vi "Exit Processing.vi"(8 "error in (no error)":errorcluster, 11 "InteractionProcessor in":refnum<class "InteractionProcessor.lvclass">) -> (0 "error out":errorcluster)   [LabVIEW 2023, in "HAF.lvlib" / "InteractionProcessor.lvclass"]
doc: "Processing will exit. Ensure a clean shutdown. All Commands are asked to cleanup which performs a controlled shutdown of Drivers."
uses:
  InteractionProcessor.lvclass
  CommandDirector/CommandDirector.lvclass
  WriteCommand/WriteCommand.lvclass
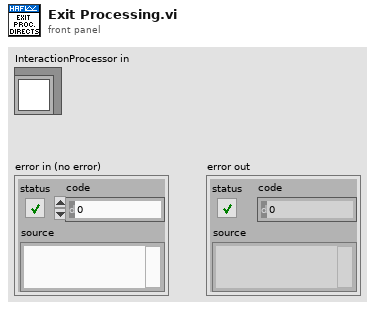
[diagram p1: front panel]
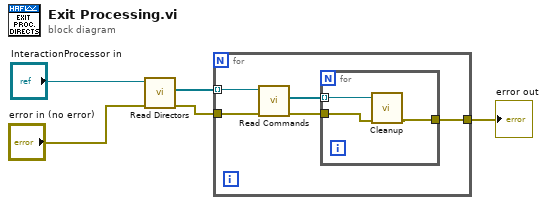
[diagram p0: block diagram]
diagram:
  n1 = call-dynamic "Read Directors.vi"("error in (no error)"="error in (no error)", "InteractionProcessor in"="InteractionProcessor in") -> ("error out"=w4:errorcluster, "Directors"=w3:refnum<class "CommandDirector.lvclass">[])  [unwired: 7 in, 1 out]
  n2 = for {
    tunnel: w3 -> [w10] mode=indexing
    tunnel: w4 -> [w9]
    tunnel: [w6] -> w5
    n3 = call-dynamic "Read Commands.vi"("error in (no error)"=w9, "CommandDirector in"=w10) -> ("error out"=w7:errorcluster, "Commands"=w8:refnum<class "WriteCommand.lvclass">[])  [unwired: 7 in, 1 out]
    n4 = for {
      tunnel: w8 -> [w13] mode=indexing
      tunnel: w7 -> [w12]
      tunnel: [w11] -> w6
      n5 = call-dynamic "Cleanup.vi"("error in (no error)"=w12, "WriteCommand in"=w13) -> ("error out"=w11:errorcluster)  [unwired: 8 in, 1 out]
    }
  }
  "error out" <- w5
